vi "loadManualToMTSUM.vi"() -> ()   [LabVIEW 2012]
uses:
  <vilib>/addons/database/Connection.llb/DB Tools Open Connec (Path).vi
  <vilib>/addons/database/Connection.llb/Conn Execute.vi
  <vilib>/addons/database/Recordset.llb/Rec Fetch Recordset Data (R).vi
  <vilib>/addons/database/Recordset.llb/Rec Destroy - Connection.vi
  <vilib>/addons/database/_DB Variant To Data/Database Variant To Data.xnode
  <vilib>/addons/database/NI_Database_API.lvlib
panel:
  out "concatenated string":string
  out "error out":errorcluster
  out "concatenated string 2":string
  in  "string":string
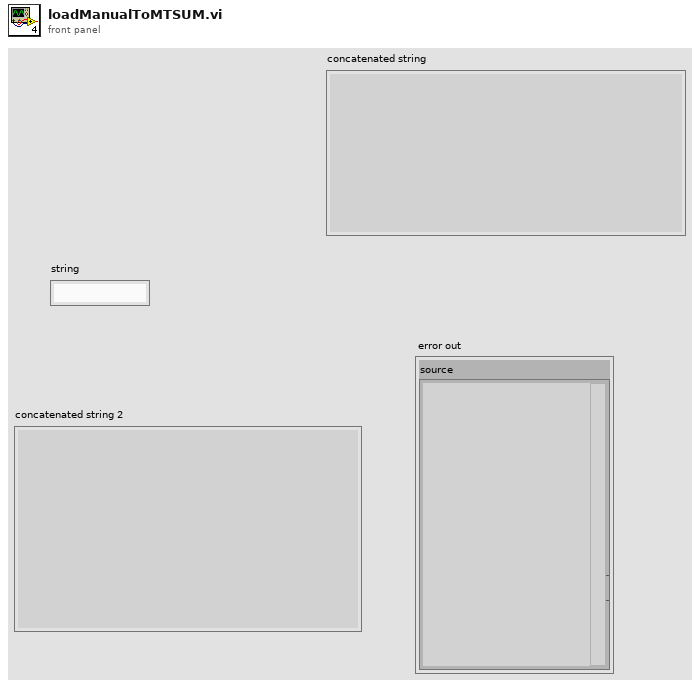
[diagram p1: front panel]
types:
  T1 = typedef "NI_Database_API.lvlib/Conn ObjectReference.ctl" = refnum<k1>
  T2 = typedef "NI_Database_API.lvlib/Rec ObjectReference.ctl" = refnum<k1>
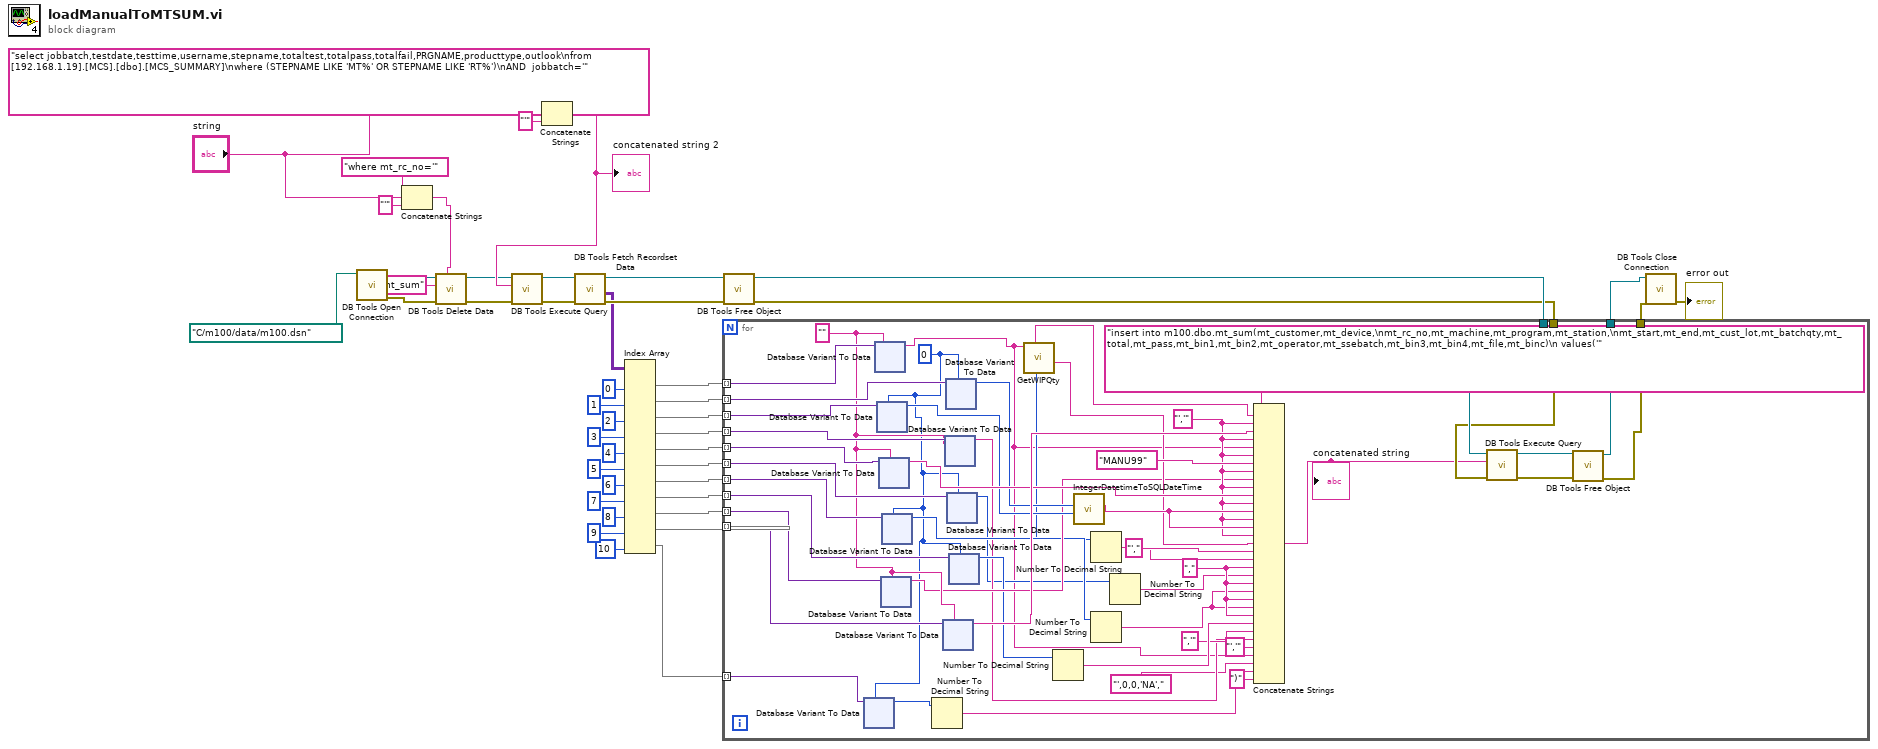
[diagram p0: block diagram]
diagram:
  n1 = call-poly <vilib>:"DB Tools Open Connection.vi"("connection information"=path "C:/m100/data/m100.dsn") -> ("error out"=w8:errorcluster, "connection reference"=w9:T1)  [unwired: 7 in]
  n2 = Concatenate Strings("where mt_rc_no='" ("string"), "string", "'" ("string")) -> (w1:string)
  n3 = call <vilib>:"DB Tools Delete Data.vi"("condition"=w1, "error in (no error)"=w8, "table"="mt_sum", "connection reference"=w9) -> ("error out"=w6:errorcluster, "connection reference out"=w7:T1)  [unwired: 6 in]
  n4 = Concatenate Strings("select jobbatch,testdate,testtime,username,stepname,totaltest,totalpass,totalfail,PRGNAME,producttype,outlook\nfrom [192.168.1.19].[MCS].[dbo].[MCS_SUMMARY]\nwhere (STEPNAME LIKE 'MT%' OR STEPNAME LIKE 'RT%')\nAND  jobbatch='" ("string"), "string", "'" ("string")) -> (w42:string)
  "concatenated string 2" <- w42
  n5 = call-poly <vilib>:"DB Tools Execute Query.vi"("error in (no error)"=w6, "SQL query"=w42, "connection reference"=w7) -> ("error out"=w39:errorcluster, "recordset reference"=w41:T2)  [unwired: 5 in]
  n6 = call-poly <vilib>:"DB Tools Fetch Recordset Data.vi"("error in (no error)"=w39, "recordset reference"=w41) -> ("error out"=w38:errorcluster, "recordset data"=w37:variant[][], "recordset reference out"=w40:T2)  [unwired: 3 in]
  n7 = Index Array(array=w37, index (col) #1=0 ("disabled index (col)"), index (col) #2=1 ("index (col)"), index (col) #3=2 ("index (col)"), index (col) #4=3 ("index (col)"), index (col) #5=4 ("index (col)"), index (col) #6=5 ("index (col)"), index (col) #7=6 ("index (col)"), index (col) #8=7 ("index (col)"), index (col) #9=8 ("index (col)"), index (col) #10=9 ("index (col)"), index (col) #11=10 ("index (col)")) -> (element #1=w27:variant[], element #2=w26:variant[], element #3=w25:variant[], element #4=w24:variant[], element #5=w23:variant[], element #6=w22:variant[], element #7=w21:variant[], element #8=w20:variant[], element #9=w19:variant[], element #10=w17:variant[], element #11=w10:variant[])  [unwired: 11 in]
  n8 = call-poly <vilib>:"DB Tools Free Object.vi"("error in (no error)"=w38, "recordset reference"=w40) -> ("error out"=w12:errorcluster, "connection reference"=w13:T1)  [unwired: 8 in]
  n9 = for {
    tunnel: w27 -> [w94] mode=indexing
    tunnel: w26 -> [w93] mode=indexing
    tunnel: w25 -> [w92] mode=indexing
    tunnel: w24 -> [w91] mode=indexing
    tunnel: w23 -> [w90] mode=indexing
    tunnel: w22 -> [w89] mode=indexing
    tunnel: w21 -> [w88] mode=indexing
    tunnel: w20 -> [w87] mode=indexing
    tunnel: w19 -> [w86] mode=indexing
    tunnel: w17 -> [w83] mode=indexing
    tunnel: [w64] -> w15
    tunnel: [w63] -> w14
    tunnel: w13 -> [w62]
    tunnel: w12 -> [w61]
    tunnel: w10 -> [w50] mode=indexing
    w68 = "," ("string")
    w74 = "','" ("string")
    w49 = 0
    w82 = ""
    n10 = xnode "Database Variant To Data"("database variant"=w50, "type"=w49) -> ("data"=w48:i32)  [unwired: 1 in, 1 out]
    n11 = xnode "Database Variant To Data"("database variant"=w94, "type"=w82) -> ("data"=w53:string)  [unwired: 1 in, 1 out]
    n12 = xnode "Database Variant To Data"("database variant"=w92, "type"=w49) -> ("data"=w77:i32)  [unwired: 1 in, 1 out]
    n13 = xnode "Database Variant To Data"("database variant"=w90, "type"=w82) -> ("data"=w79:string)  [unwired: 1 in, 1 out]
    n14 = xnode "Database Variant To Data"("database variant"=w86, "type"=w82) -> ("data"=w72:string)  [unwired: 1 in, 1 out]
    n15 = xnode "Database Variant To Data"("database variant"=w88, "type"=w49) -> ("data"=w70:i32)  [unwired: 1 in, 1 out]
    n16 = Number To Decimal String(number=w48) -> (decimal integer string=w47:string)  [unwired: 1 in]
    n17 = xnode "Database Variant To Data"("database variant"=w83, "type"=w82) -> ("data"=w81:string)  [unwired: 1 in, 1 out]
    n18 = xnode "Database Variant To Data"("database variant"=w91, "type"=w82) -> ("data"=w58:string)  [unwired: 1 in, 1 out]
    n19 = xnode "Database Variant To Data"("database variant"=w93, "type"=w49) -> ("data"=w78:i32)  [unwired: 1 in, 1 out]
    n20 = xnode "Database Variant To Data"("database variant"=w89, "type"=w49) -> ("data"=w55:i32)  [unwired: 1 in, 1 out]
    n21 = xnode "Database Variant To Data"("database variant"=w87, "type"=w49) -> ("data"=w69:i32)  [unwired: 1 in, 1 out]
    n22 = call "GetWIPQty.vi"("Lotno"=w53) -> ("lotno"=w75:string, "BATCHQTY"=w57:i32, "CustomerID"=w84:string)  [unwired: 2 in, 6 out]
    n23 = Number To Decimal String(number=w69) -> (decimal integer string=w67:string)  [unwired: 1 in]
    n24 = call "IntegerDatetimeToSQLDateTime.vi"("Time"=w77, "Date"=w78) -> ("SQL Datime"=w76:string)  [unwired: 9 in]
    n25 = Number To Decimal String(number=w57) -> (decimal integer string=w71:string)  [unwired: 1 in]
    n26 = Number To Decimal String(number=w70) -> (decimal integer string=w54:string)  [unwired: 1 in]
    n27 = Number To Decimal String(number=w55) -> (decimal integer string=w56:string)  [unwired: 1 in]
    n28 = Concatenate Strings("insert into m100.dbo.mt_sum(mt_customer,mt_device,\nmt_rc_no,mt_machine,mt_program,mt_station,\nmt_start,mt_end,mt_cust_lot,mt_batchqty,mt_total,mt_pass,mt_bin1,mt_bin2,mt_operator,mt_ssebatch,mt_bin3,mt_bin4,mt_file,mt_binc)\n values('" ("string"), w84, w74, w81, w74, w53, w74, "MANU99" ("string"), w74, w72, w74, w79, w74, w76, w74, w76, w74, w75, "'," ("string"), w71, w68, w56, w68, w54, w68, w54, w68, w67, ",'" ("string"), w58, "','" ("string"), w53, "',0,0,'NA'," ("string"), w47, ")" ("string")) -> (w60:string)
    "concatenated string" <- w60
    n29 = call-poly <vilib>:"DB Tools Execute Query.vi"("error in (no error)"=w61, "SQL query"=w60, "connection reference"=w62) -> ("error out"=w65:errorcluster, "recordset reference"=w66:T2)  [unwired: 5 in]
    n30 = call-poly <vilib>:"DB Tools Free Object.vi"("error in (no error)"=w65, "recordset reference"=w66) -> ("error out"=w63:errorcluster, "connection reference"=w64:T1)  [unwired: 8 in]
  }
  n31 = call <vilib>:"DB Tools Close Connection.vi"("error in (no error)"=w14, "connection reference"=w15) -> ("error out"=→"error out":errorcluster)  [unwired: 5 in]
